vi "NI VeriStand - Get Multiple Alarms Data.vi"(7 "Target":string, 8 "error in (no error)":errorcluster, 9 "timeout (ms)":u32=10000, 10 "Alarm Names":string[](array[string]), 11 "AlarmManager in":T2) -> (0 "error out":errorcluster, 2 "Alarms Data":T1[](array[typedef]) {"Trip Value" format="%.2f"; "Delay" format="%.2f"; "Low Limit" format="%.2f"; "High Limit" format="%.2f"}, 3 "AlarmManager out":T2)   [LabVIEW 2020, in "NI_VS AlarmManager ExecutionAPI.lvlib"]
doc: "Returns high limit, low limit, corresponding procedure name, delay duration, trip value, priority, state, mode, group number, priority number, name, and full name information about the alarms you specify."
uses:
  <vilib>/NI VeriStand/Execution/AlarmManager/NI_VS AlarmManager ExecutionAPI.lvlib
  <vilib>/NI VeriStand/Execution/AlarmManager/AlarmManagerAPI.ctl
  NationalInstruments.VeriStand.ClientAPI
  <vilib>/NI VeriStand/Execution/Alarm/AlarmInfo.ctl
  <vilib>/NI VeriStand/Execution/Alarm/NI_VS Alarm ExecutionAPI.lvlib
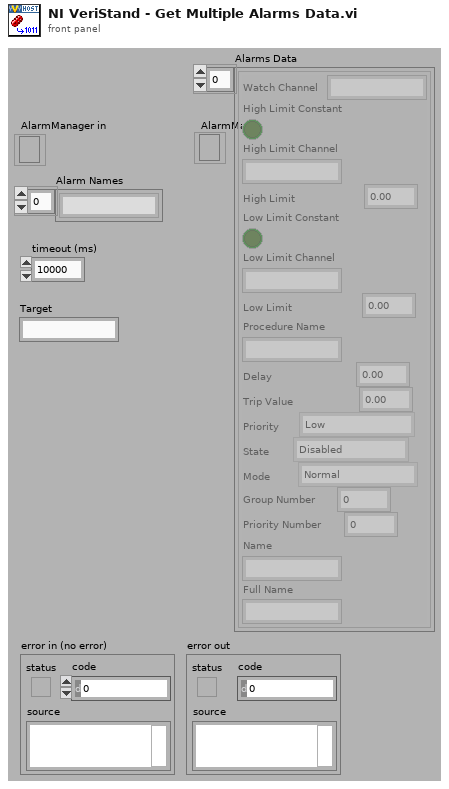
[diagram p1: front panel]
types:
  T1 = typedef "NI_VS Alarm ExecutionAPI.lvlib/AlarmInfo.ctl" = cluster{"Watch Channel":string, "High Limit Constant":bool, "High Limit Channel":string, "High Limit":dbl, "Low Limit Constant":bool, "Low Limit Channel":string, "Low Limit":dbl, "Procedure Name":string, "Delay":dbl, "Trip Value":dbl, "Priority":enum16{"Low", "Medium", "High"}, "State":enum16{"Disabled", "Enabled", "Tripped", "Delayed Trip", "Indicate"}, "Mode":enum16{"Normal", "Indicate Only"}, "Group Number":u32, "Priority Number":u32, "Name":string, "Full Name":string}
  T2 = typedef "NI_VS AlarmManager ExecutionAPI.lvlib/AlarmManagerAPI.ctl" = refnum<k24>
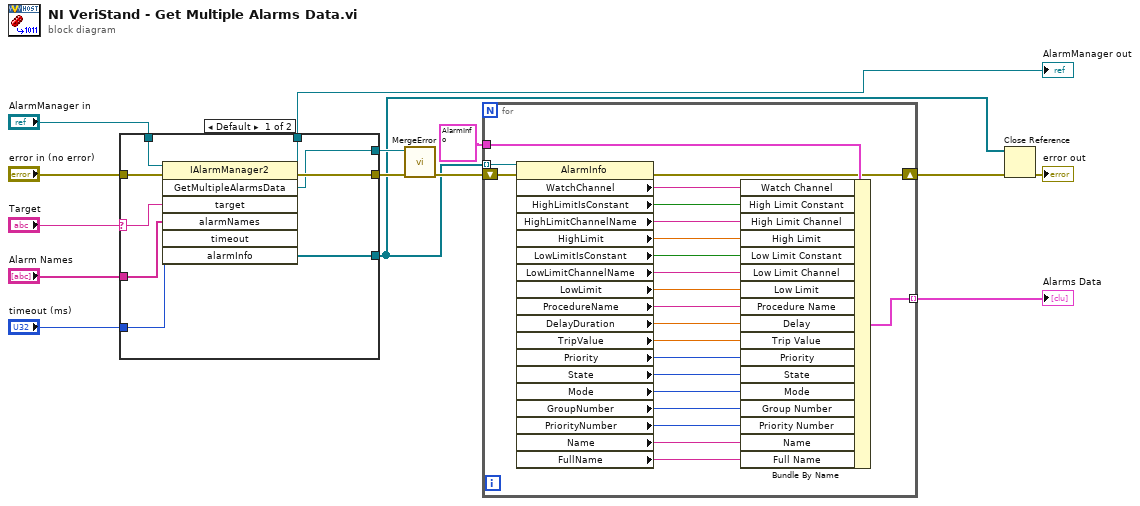
[diagram p0: block diagram]
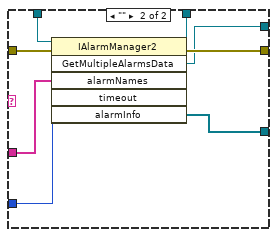
[diagram p2: hidden frame]
diagram:
  n1 = case shown="Default" "Target" {
    selector: "Target" -> [w15 _]
    tunnel: "AlarmManager in" -> [w23 w31]
    tunnel: [w22 w30] -> w13
    tunnel: [w21 w29] -> w12
    tunnel: [w20 w28] -> w11
    tunnel: "error in (no error)" -> [w19 w27]
    tunnel: "Alarm Names" -> [w18 w26]
    tunnel: "timeout (ms)" -> [w17 w25]
    tunnel: [w16 w24] -> w1
    frame Default {
      n2 = invoke class="IAlarmManager2" method="GetMultipleAlarmsData"(reference=w23, error in=w19, "target"=w15, "alarmNames"=w18, "timeout"=w17) -> (reference out=w22:T2, error out=w21:errorcluster, "GetMultipleAlarmsData"=w20:refnum<k24>, "alarmInfo"=w16:refnum<k24>[])  [unwired: 2 in, 3 out]
    }
    frame "" {
      n3 = invoke class="IAlarmManager2" method="GetMultipleAlarmsData"(reference=w31, error in=w27, "alarmNames"=w26, "timeout"=w25) -> (reference out=w30:T2, error out=w29:errorcluster, "GetMultipleAlarmsData"=w28:refnum<k24>, "alarmInfo"=w24:refnum<k24>[])  [unwired: 2 in, 2 out]
    }
  }
  "AlarmManager out" <- w13
  n4 = call <vilib>:"MergeError.vi"("error in (no error)"=w12, "Error"=w11) -> ("error out"=w9:errorcluster)  [unwired: 9 out]
  n5 = for {
    tunnel: w1 -> [w40] mode=indexing
    shift-right: [w35] -> w8
    shift-left: w9 -> [w39]
    tunnel: [w38] -> w5 mode=indexing
    tunnel: T1 {"Watch Channel"="", "High Limit Constant"=FALSE, "High Limit Channel"="", "High Limit"=0.0, "Low Limit Constant"=FALSE, "Low Limit Channel"="", "Low Limit"=0.0, "Procedure Name"="", "Delay"=0.0, "Trip Value"=0.0, "Priority"=enum."Low", "State"=enum."Disabled", "Mode"=enum."Normal", "Group Number"=0, "Priority Number"=0, "Name"="", "Full Name"=""} ("AlarmInfo") -> [w37]
    n6 = property class="AlarmInfo"(reference=w40, error in=w39) -> (error out=w35:errorcluster, "WatchChannel"=w53:string, "HighLimitIsConstant"=w52:bool, "HighLimitChannelName"=w51:string, "HighLimit"=w50:dbl, "LowLimitIsConstant"=w49:bool, "LowLimitChannelName"=w48:string, "LowLimit"=w47:dbl, "ProcedureName"=w46:string, "DelayDuration"=w45:dbl, "TripValue"=w44:dbl, "Priority"=w43:u8, "State"=w42:u8, "Mode"=w41:u8, "GroupNumber"=w36:u32, "PriorityNumber"=w34:u32, "Name"=w33:string, "FullName"=w32:string)  [unwired: 1 out]
    n7 = Bundle By Name(cluster=w37, "Watch Channel"=w53, "High Limit Constant"=w52, "High Limit Channel"=w51, "High Limit"=w50, "Low Limit Constant"=w49, "Low Limit Channel"=w48, "Low Limit"=w47, "Procedure Name"=w46, "Delay"=w45, "Trip Value"=w44, "Priority"=w43, "State"=w42, "Mode"=w41, "Group Number"=w36, "Priority Number"=w34, "Name"=w33, "Full Name"=w32) -> (w38:T1)
  }
  "Alarms Data" <- w5
  n8 = Close Reference(reference=w1, error in (no error)=w8) -> (error out=→"error out":errorcluster)
